vi "client.vi"() -> ()   [LabVIEW 2019]
uses:
  Generated_client/RPC Messages/Greeter_Color.ctl
  Generated_client/RPC Messages/Greeter_req.ctl
  Generated_client/RPC Messages/Greeter_req_req_oneof/Greeter_req_req_oneof.lvclass
  Generated_client/RPC Messages/Greeter_req_req_oneof/Greeter_req_req_oneof.lvclass/Greeter_req_req_oneof.ctl
  Generated_client/RPC Messages/Greeter_res_res_oneof/Greeter_res_res_oneof.lvclass/Greeter_res_res_oneof.ctl
  Generated_client/Generated_client.lvlib
  Generated_client/RPC Messages/Greeter_res_res_oneof/Greeter_res_res_oneof.lvclass
panel:
  out "res_name":string
  out "res_color":T1
  out "res_latitude":i32
  in  "req_latitude":i32
  in  "req_color":T1
  in  "req_name":string
  in  "Enum":enum16{"req_name", "req_color"}(ring)
  out "error out":errorcluster
  in  "error in":errorcluster
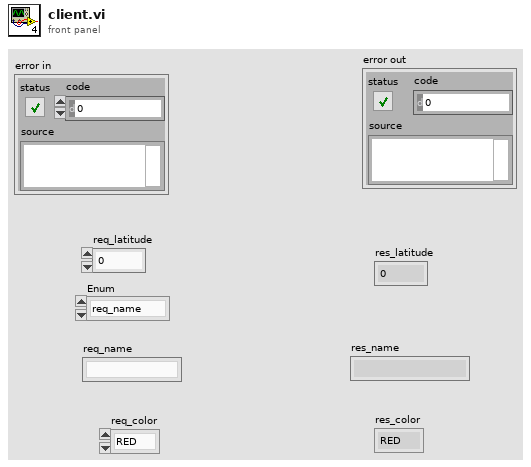
[diagram p1: front panel]
types:
  T1 = typedef "Generated_client.lvlib/Greeter_Color.ctl" = enum32{"RED", "GREEN", "BLUE"}
  T2 = typedef "Generated_client.lvlib/Greeter_req.ctl" = cluster{"req_latitude":i32, "Greeter_req_req_oneof":refnum<class "Greeter_req_req_oneof.lvclass">}
  T3 = typedef "grpc-lvsupport-release.lvlib/grpcId.ctl" = u64
  T4 = typedef "Generated_client.lvlib/Greeter_res.ctl" = cluster{"res_latitude":i32, "Greeter_res_res_oneof":refnum<class "Greeter_res_res_oneof.lvclass">}
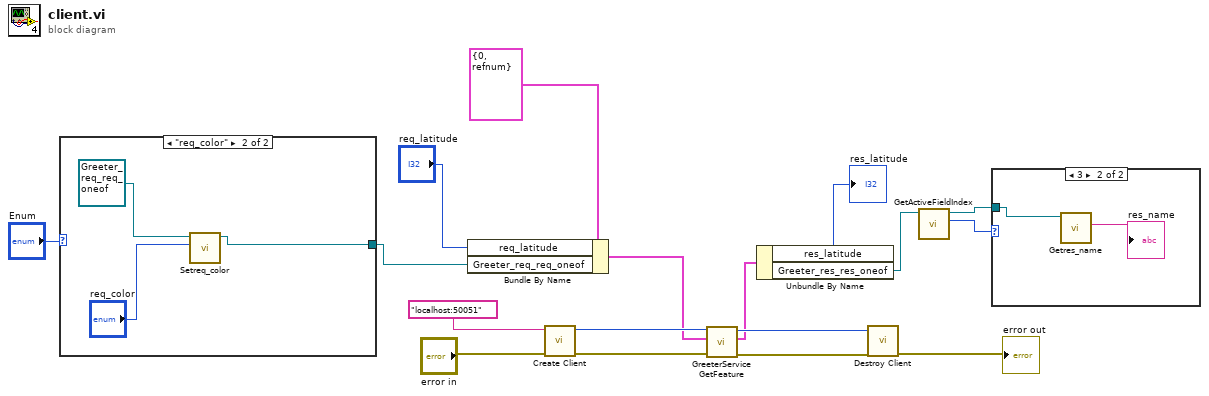
[diagram p0: block diagram]
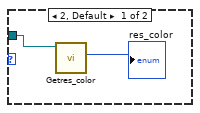
[diagram p2: hidden frame]
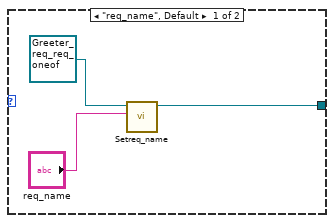
[diagram p3: hidden frame]
diagram:
  n1 = case shown="\"req_color\"" "Enum" {
    tunnel: [w18 w21] -> w8
    frame "req_name", Default {
      n2 = call "Setreq_name.vi"("Set_Val"="req_name", "OneOfTemplate in"=refnum<class "Greeter_req_req_oneof.lvclass"> refnum) -> ("OneOfTemplate out"=w18:refnum<class "Greeter_req_req_oneof.lvclass">)  [unwired: 8 in, 1 out]
    }
    frame "req_color" {
      n3 = call "Setreq_color.vi"("Set_Val"="req_color", "OneOfTemplate in"=refnum<class "Greeter_req_req_oneof.lvclass"> refnum) -> ("OneOfTemplate out"=w21:refnum<class "Greeter_req_req_oneof.lvclass">)  [unwired: 8 in, 1 out]
    }
  }
  n4 = Bundle By Name(cluster=T2 {"req_latitude"=0, "Greeter_req_req_oneof"=refnum} ("Greeter_req"), "req_latitude"="req_latitude", "Greeter_req_req_oneof"=w8) -> (w7:T2)
  n5 = call "Create Client.vi"("error in"="error in", "address"="localhost:50051") -> ("error out"=w15:errorcluster, "gRPC ID Out"=w17:T3)  [unwired: 8 in]
  n6 = call "GreeterService GetFeature.vi"("error in"=w15, "Request Data"=w7, "gRPC ID"=w17) -> ("error out"=w14:errorcluster, "Response Data"=w6:T4, "gRPC ID out"=w16:T3)  [unwired: 6 in]
  n7 = Unbundle By Name(w6) -> ("res_latitude"=→"res_latitude":i32, "Greeter_res_res_oneof"=w4:refnum<class "Greeter_res_res_oneof.lvclass">)
  n8 = call "Destroy Client.vi"("error in"=w14, "gRPC ID"=w16) -> ("error out"=→"error out":errorcluster)  [unwired: 9 in]
  n9 = call "GetActiveFieldIndex.vi"("OneOfTemplate in"=w4) -> ("Active Field Index"=w3:i32, "OneOfTemplate out"=w2:refnum<class "Greeter_res_res_oneof.lvclass">)  [unwired: 8 in, 1 out]
  n10 = case shown="3" w3 {
    tunnel: w2 -> [w25 w27]
    frame 2, Default {
      n11 = call "Getres_color.vi"("OneOfTemplate in"=w25) -> ("Get_Val"=→"res_color":T1)  [unwired: 8 in, 2 out]
    }
    frame 3 {
      n12 = call "Getres_name.vi"("OneOfTemplate in"=w27) -> ("Get_Val"=→"res_name":string)  [unwired: 8 in, 2 out]
    }
  }
